vi "K_S30_VISA F33.vi"(4 "error in":errorcluster, 5 "Configuration":u8, 6 "Config. Nr.":u8, 7 "Address":u8=250) -> (0 "error out":errorcluster)   [LabVIEW 2012]
panel:
  # "Function 30: Write configuration\nV1.0, b.v."
  # "Attention!\nPlease read carefully the documentation for this\nfunction.\nSome configuration Bytes are as nibble, some as Flags!\nReadout first the config. Byte before you modify it."
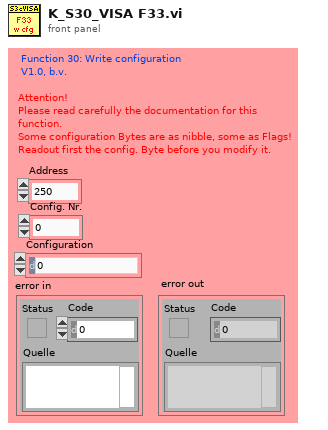
[diagram p1: front panel]
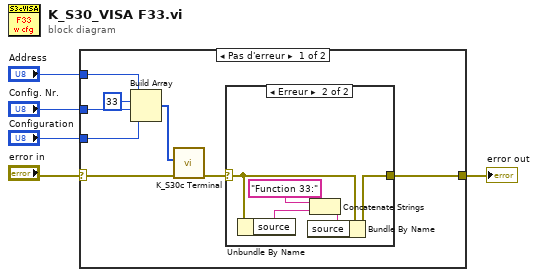
[diagram p0: block diagram]
diagram:
  n1 = case shown="Pas d'erreur" "error in" {
    selector: "error in" -> [w10 w20]
    tunnel: "Address" -> [w13 _]
    tunnel: [w8 w20] -> w3
    tunnel: "Config. Nr." -> [w7 _]
    tunnel: "Configuration" -> [w6 _]
    frame No Error {
      n2 = Build Array(w13, u8 33 ("Element"), w7, w6) -> (w11:u8[])
      n3 = call "K_S30c Terminal.vi"("error in"=w10, "request"=w11) -> ("error out"=w9:errorcluster)  [unwired: 4 in, 1 out]
      n4 = case shown="Erreur" w9 {
        selector: w9 -> [w14 w19]
        tunnel: [w14 w17] -> w8
        frame No Error {
        }
        frame Error {
          n5 = Unbundle By Name(w19) -> ("source"=w16:string)
          n6 = Concatenate Strings("Function 33:" ("String"), w16) -> (w18:string)
          n7 = Bundle By Name(cluster=w19, "source"=w18) -> (w17:errorcluster)
        }
      }
    }
    frame Error {
    }
  }
  "error out" <- w3
